vi "Front Panel.vi"() -> ()   [LabVIEW 2020]
uses:
  XControl/Step Control/Step.xctl
  Function/Copy of Function Folder/Function V3.lvlib
panel:
  out "Running?":bool
  in  "Information":string
  in  "File Counter":i32
  in  "Data File Destination":path
  in  "Autorun":bool
  in  "Browser":enum32{"Scan", "Read", "Array"}(tab)
  out "Scan Process Preview":T1(array[cluster]) {"Scan Instrument" items=["Keithley 6430 Scan Voltage", "Dynacool SetField 100Oe", "Dynacool SetPosition", "Dynacool SetTemperature hold", "Dynacool SetTemperature no hold", "Read Time(s)"]}
  out "Read Process Preview":u16[](array[ring]) items=["Keithley 6430 Read Current", "Keithley 6430 Read Voltage", "Dynacool Ch1", "Dynacool Ch2", "Dynacool Ch3", "Dynacool GetField", "Dynacool GetTemperature", "Dynacool GetPosition", "Read Secs"]
  in  "Preview":bool
  in  "Array Preview":string[][](table)
  in  "Step":T2(xcontrol)
  in  "Start":bool
  in  "Load Configuration":bool
  in  "INI File Destination":path
  in  "Read Instrument":i32(listbox)
  in  "Scan Instrument":i32(listbox)
  in  "Initialize":bool
  in  "Quit":bool
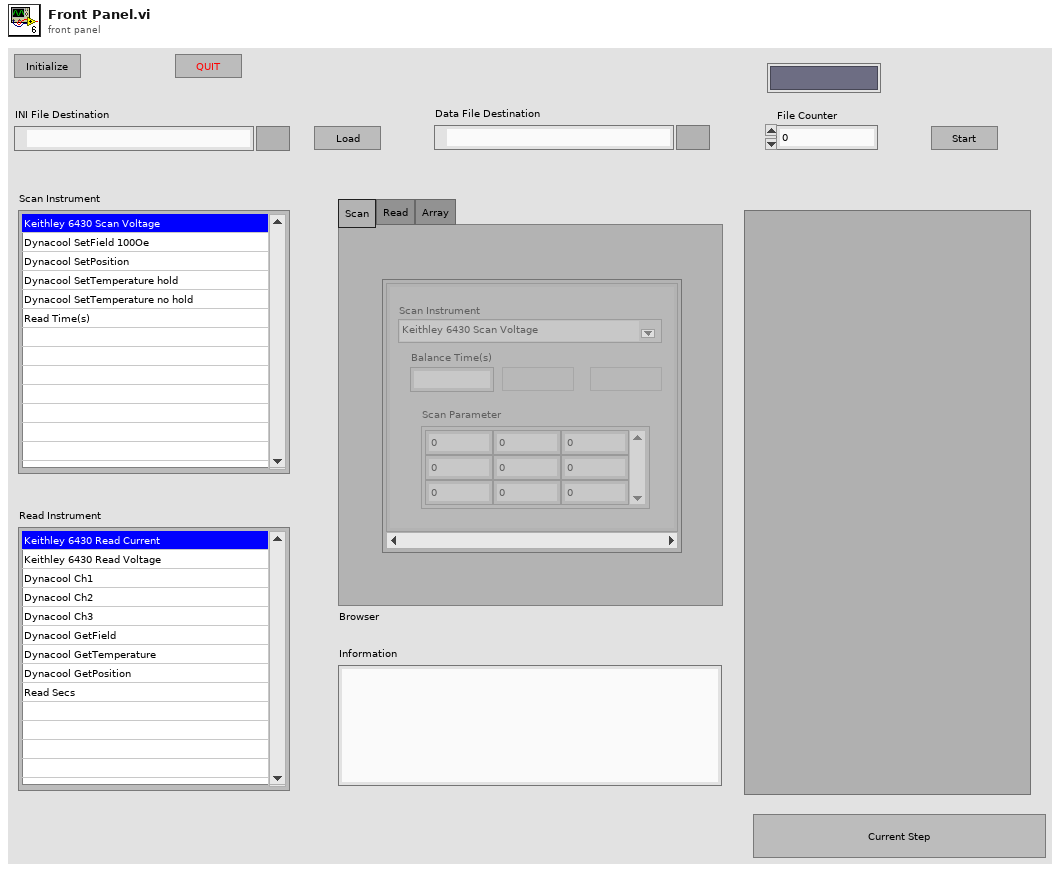
[diagram p1: front panel]
types:
  T1 = cluster{"Scan Instrument":u16, "Linear/Log":bool, "Period/Number":bool, "Balance Time(s)":dbl, "Scan Parameter":dbl[][]}[]
  T2 = cluster{"Wait(s)":dbl, "Interplate Method":u16, "Read Process":u16[], "Scan Process":cluster{"Scan Instrument":u16, "Linear/Log":bool, "Period/Number":bool, "Balance Time(s)":dbl, "Scan Parameter":dbl[][]}[], "Step Information":cluster{"Step Name":string, "Step Description":string}}[]
  T3 = enum16{"Initialize", "Load Configuration", "Preview", "Start", "Shutdown"}
  T4 = cluster{"Wait(s)":dbl, "Interplate Method":u16, "Read Process":u16[], "Scan Process":cluster{"Scan Instrument":u16, "Linear/Log":bool, "Period/Number":bool, "Balance Time(s)":dbl, "Scan Parameter":dbl[][]}[], "Step Information":cluster{"Step Name":string, "Step Description":string}}
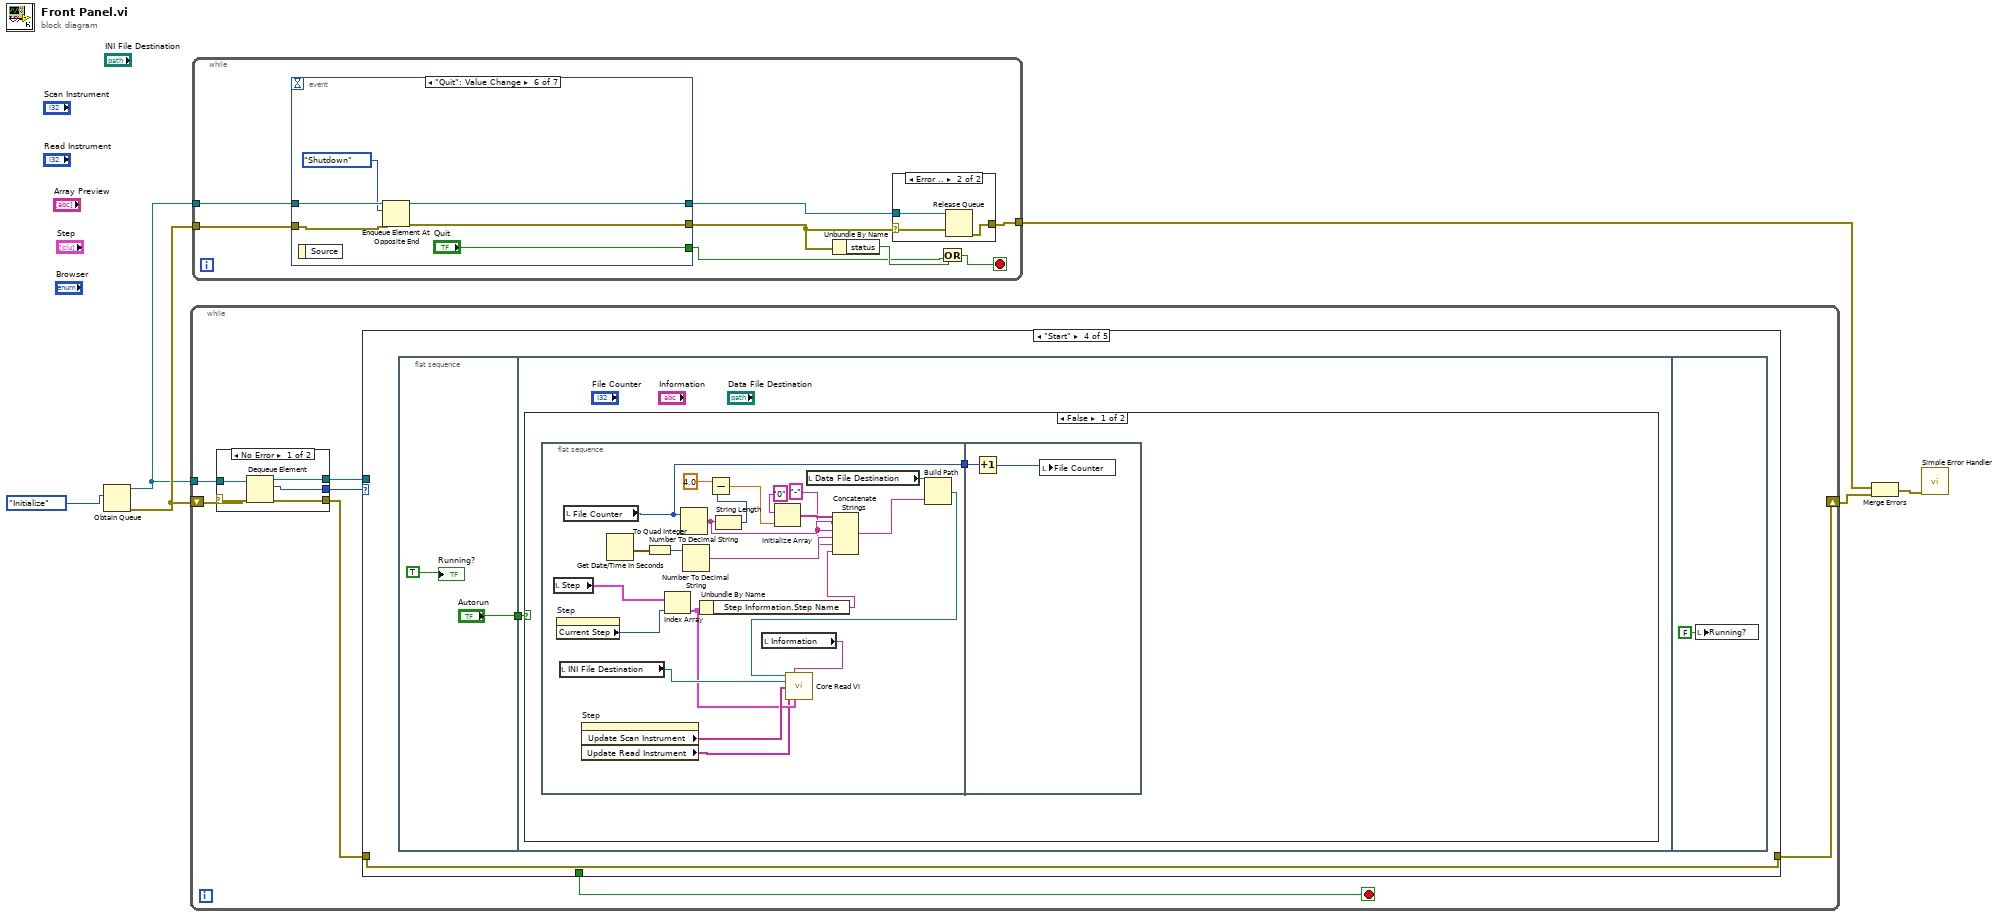
[diagram p0: block diagram]
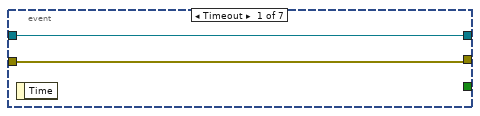
[diagram p3: hidden frame]
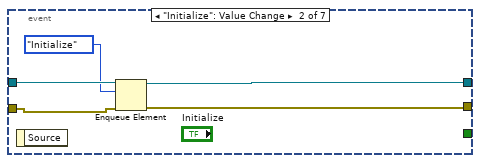
[diagram p4: hidden frame]
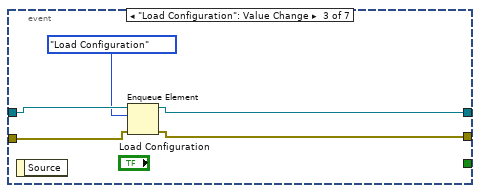
[diagram p5: hidden frame]
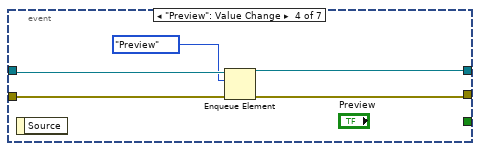
[diagram p6: hidden frame]
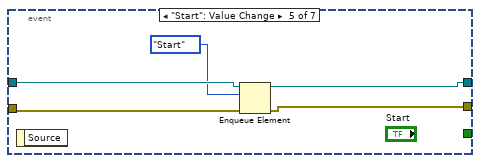
[diagram p7: hidden frame]
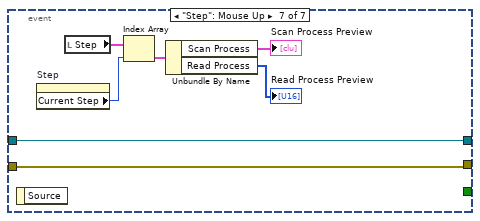
[diagram p8: hidden frame]
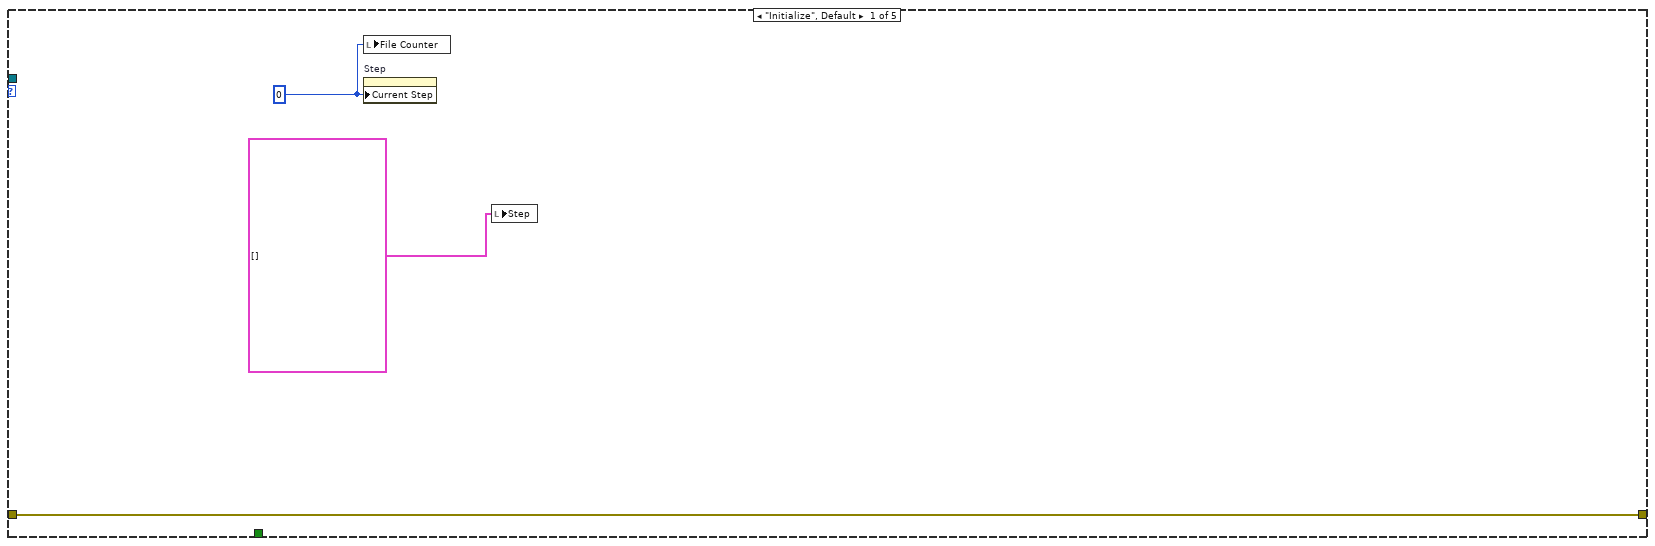
[diagram p9: hidden frame]
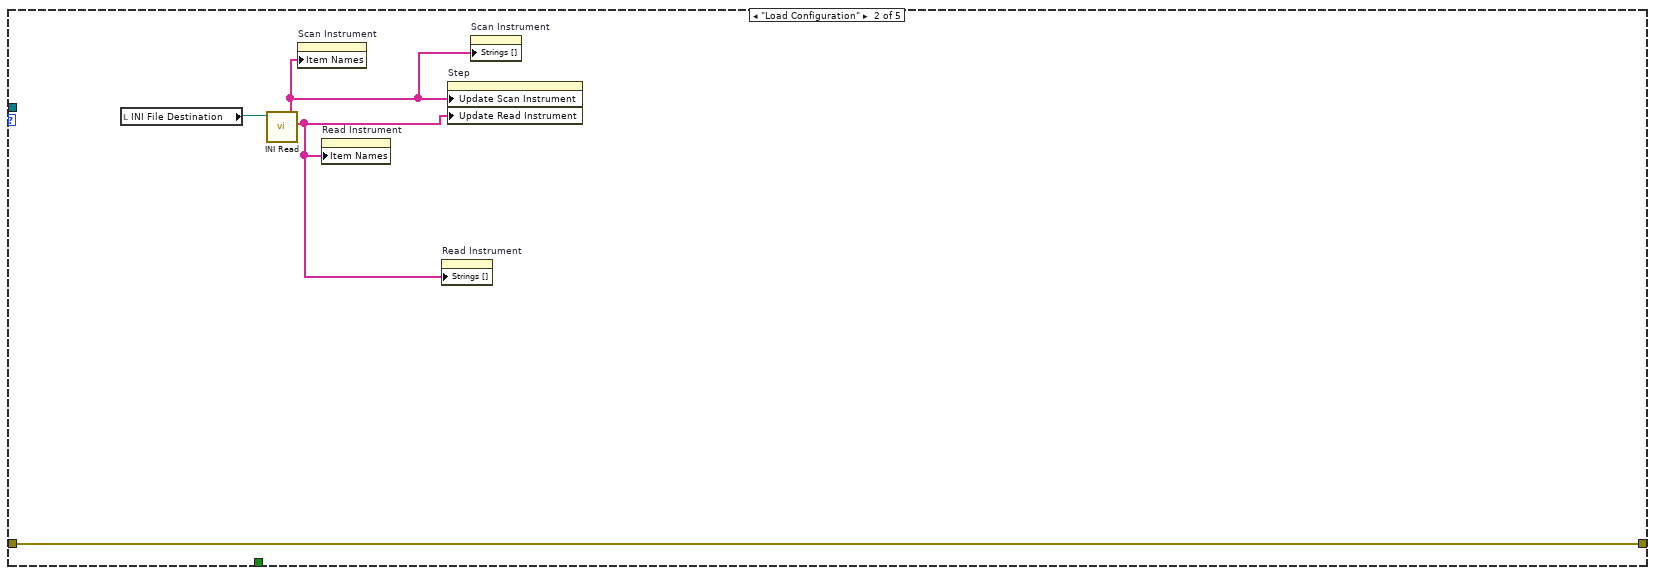
[diagram p10: hidden frame]
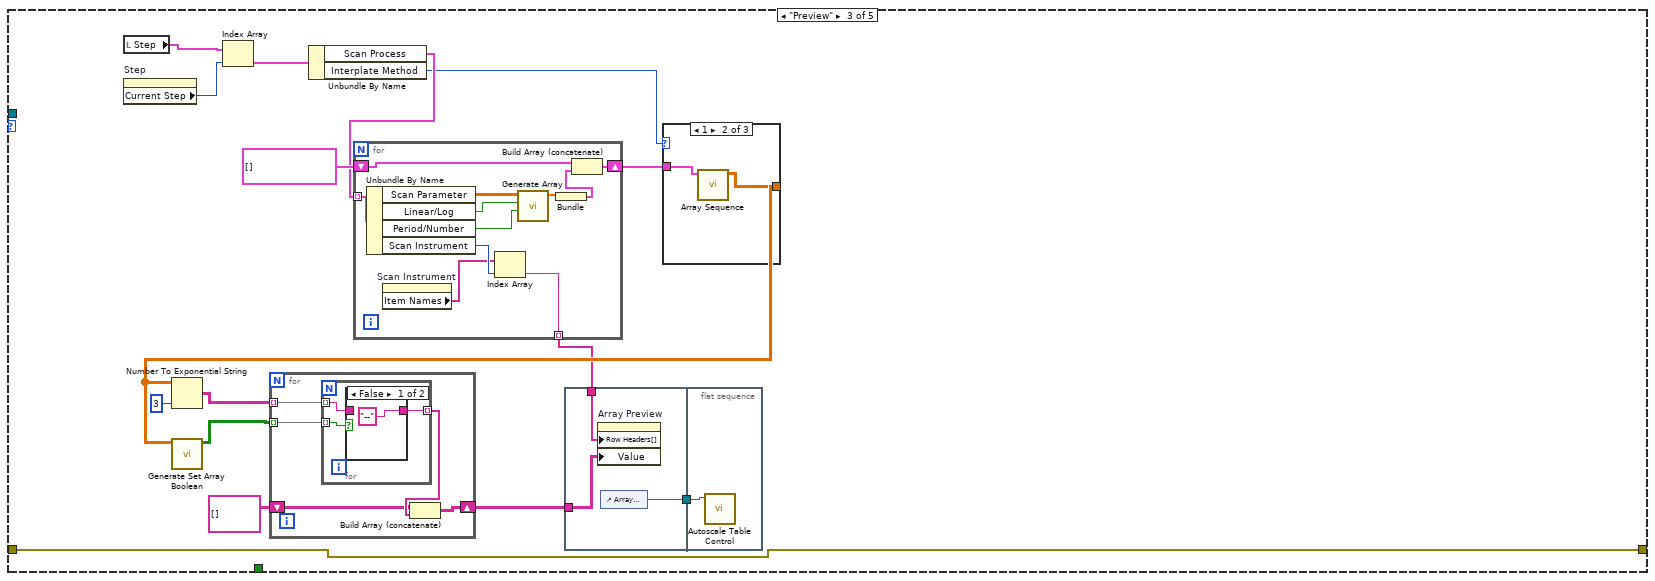
[diagram p11: hidden frame]
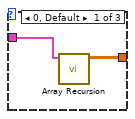
[diagram p13: hidden frame]
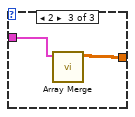
[diagram p14: hidden frame]
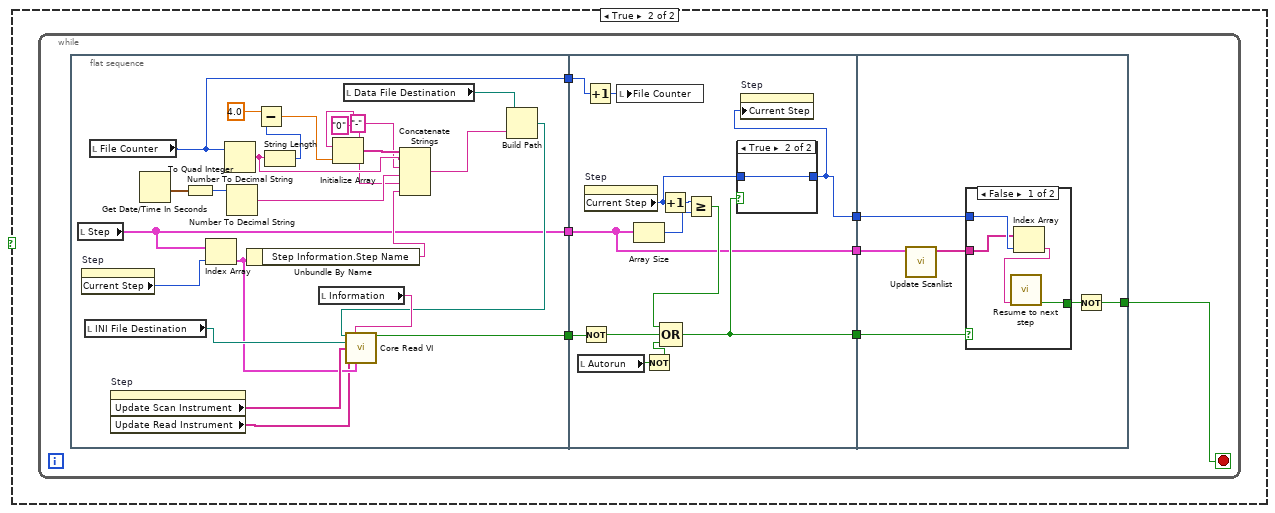
[diagram p15: hidden frame]
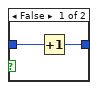
[diagram p16: hidden frame]
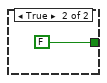
[diagram p17: hidden frame]
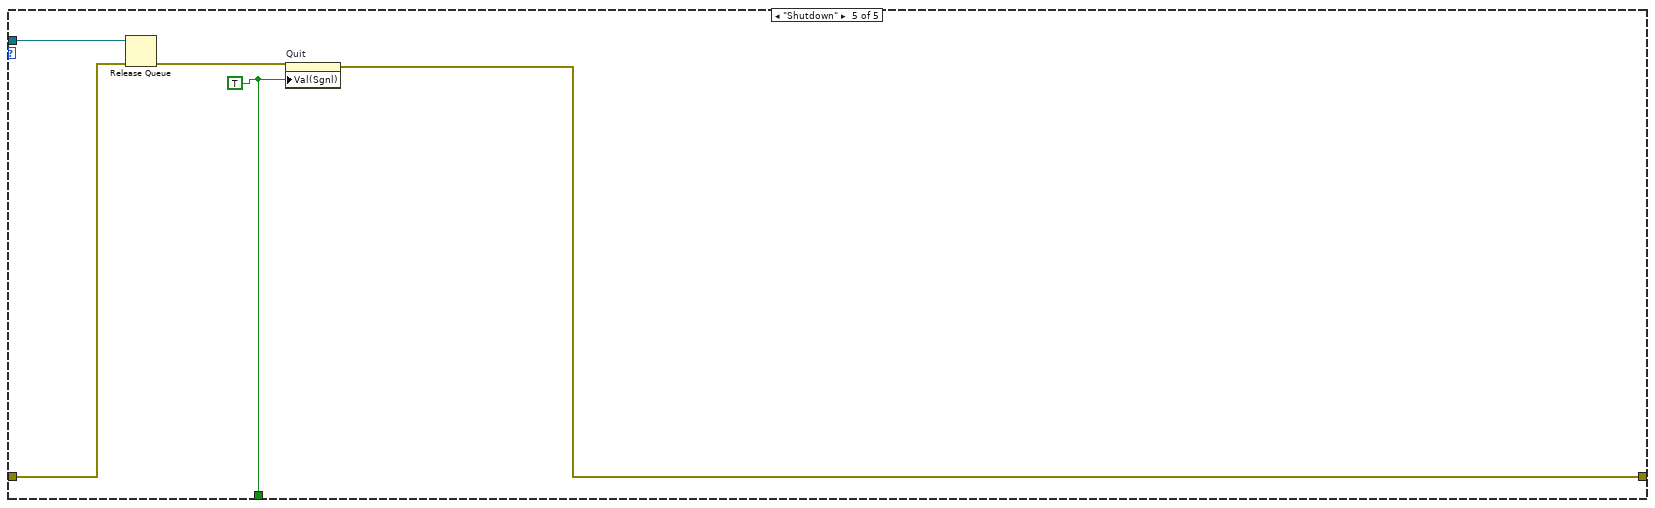
[diagram p18: hidden frame]
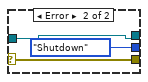
[diagram p19: hidden frame]
diagram:
  n1 = Obtain Queue(element data type=T3."Initialize" ("element")) -> (queue out=w5:refnum<queue>, error out=w6:errorcluster)  [unwired: 4 in, 1 out]
  n2 = while {
    shift-right: [w7] -> w4
    shift-left: w6 -> [w13]
    tunnel: w5 -> [w12]
    stop <- w10 stop-if-true
    n3 = case shown="No Error" w13 {
      selector: w13 -> [w165 w168]
      tunnel: [w164 w168] -> w9
      tunnel: w12 -> [w163 w167]
      tunnel: [w162 w167] -> w11
      tunnel: [w161 T3."Shutdown" ("element")] -> w8
      frame No Error {
        n4 = Dequeue Element(queue=w163, error in (no error)=w165) -> (queue out=w162:refnum<queue>, element=w161:T3, error out=w164:errorcluster)  [unwired: 1 in, 1 out]
      }
      frame Error {
      }
    }
    n5 = case shown="\"Start\"" w8 {
      tunnel: w11 -> [_ _ _ _ w159]
      tunnel: w9 -> [w16 w17 w21 w69 w160]
      tunnel: [w16 w17 w21 w69 w157] -> w7
      tunnel: [_ _ _ _ w156] -> w10
      frame "Initialize", Default {
        w14 = 0 ("Current Step")
        n6 = local write "File Counter"(w14) -> ()
        n7 = property on="Step" class="Step (strict)"("Current Step"=w14) -> ()  [unwired: 2 in, 2 out]
        n8 = local write "Step"(T2 []) -> ()
      }
      frame "Load Configuration" {
        n9 = local read "INI File Destination"() -> (w20:path)
        n10 = call "INI Read.vi"("configuration file path"=w20) -> ("Read Instrument String"=w19:string[], "Scan Instrument String"=w18:string[])  [unwired: 7 in, 2 out]
        n11 = property on="Scan Instrument" class="LstBox (strict)"("Item Names"=w18) -> ()  [unwired: 2 in, 2 out]
        n12 = property on="Read Instrument" class="LstBox (strict)"("Item Names"=w19) -> ()  [unwired: 2 in, 2 out]
        n13 = property on="Read Instrument" class="Ring (strict)"("Strings []"=w19) -> ()  [unwired: 2 in, 2 out]
        n14 = property on="Step" class="Step (strict)"("Update Scan Instrument"=w18, "Update Read Instrument"=w19) -> ()  [unwired: 2 in, 2 out]
        n15 = property on="Scan Instrument" class="Ring (strict)"("Strings []"=w18) -> ()  [unwired: 2 in, 2 out]
      }
      frame "Preview" {
        n16 = local read "Step"() -> (w35:T2)
        n17 = property on="Step" class="Step (strict)"() -> ("Current Step"=w36:i32)  [unwired: 2 in, 2 out]
        n18 = Index Array(array=w35, index=w36) -> (element=w34:T4)
        n19 = Unbundle By Name(w34) -> ("Scan Process"=w32:T1, "Interplate Method"=w31:u16)
        n20 = for {
          tunnel: w32 -> [w67] mode=indexing
          shift-right: [w65] -> w30
          shift-left: cluster{"Output":dbl[]}[] [] -> [w64]
          tunnel: [w62] -> w24 mode=indexing
          n21 = Unbundle By Name(w67) -> ("Scan Parameter"=w60:dbl[][], "Linear/Log"=w59:bool, "Period/Number"=w58:bool, "Scan Instrument"=w63:u16)
          n22 = property on="Scan Instrument" class="LstBox (strict)"() -> ("Item Names"=w57:string[])  [unwired: 2 in, 2 out]
          n23 = Index Array(array=w57, index=w63) -> (element=w62:string)
          n24 = call "Generate Array.vi"("Period/Number"=w58, "Linear/Log"=w59, "Input Array"=w60) -> ("Output"=w61:dbl[])  [unwired: 8 in]
          n25 = Bundle("Output"=w61) -> (w66:cluster{"Output":dbl[]})  [unwired: 1 in]
          n26 = Build Array (concatenate)(w64, w66) -> (w65:cluster{"Output":dbl[]}[])
        }
        n27 = flat-sequence {
          tunnel: w24 -> [w39]
          tunnel: w23 -> [w38]
          tunnel: [w37] -> w22
          tunnel: w22 -> [w40]
          frame #0 {
            n28 = property on="Array Preview" class="Tbl (strict)"("Row Headers[]"=w39, "Value"=w38) -> ()  [unwired: 2 in, 2 out]
            n29 = control-ref of="Array Preview"() -> (w37:refnum<vi>)
          }
          frame #1 {
            n30 = call "Autoscale Table Control.vi"("Input Table Control"=w40) -> ()  [unwired: 10 in, 1 out]
          }
        }
        n31 = case shown="1" w31 {
          tunnel: w30 -> [w52 w54 w56]
          tunnel: [w51 w53 w55] -> w29
          frame 0, Default {
            n32 = call "Array Recursion.vi"("Input Cluster Array"=w52) -> ("Output Array"=w51:dbl[][])  [unwired: 10 in]
          }
          frame 1 {
            n33 = call "Array Sequence.vi"("Input Cluster Array"=w54) -> ("Output Sequence Array"=w53:dbl[][])  [unwired: 10 in]
          }
          frame 2 {
            n34 = call "Array Merge.vi"("Input Cluster Array"=w56) -> ("Output Array"=w55:dbl[][])  [unwired: 10 in]
          }
        }
        n35 = Number To Exponential String(number=w29, precision (6)=i16 3) -> (E-format string=w26:string[][])  [unwired: 2 in]
        n36 = call "Generate Set Array Boolean.vi"("Input Array"=w29) -> ("Output Bool Array"=w25:bool[][])  [unwired: 10 in]
        n37 = for {
          tunnel: w26 -> [w44] mode=indexing
          tunnel: w25 -> [w45] mode=indexing
          shift-right: [w42] -> w23
          shift-left: string[][] [] -> [w41]
          n38 = for {
            tunnel: w45 -> [w48] mode=indexing
            tunnel: w44 -> [w47] mode=indexing
            tunnel: [w46] -> w43 mode=indexing
            n39 = case shown="False" w48 {
              tunnel: w47 -> [_ w50]
              tunnel: ["--" w50] -> w46
              frame False {
              }
              frame True {
              }
            }
          }
          n40 = Build Array (concatenate)(w41, w43) -> (w42:string[][])
        }
      }
      frame "Start" {
        n41 = flat-sequence {
          tunnel: ["Autorun"] -> w68
          tunnel: w68 -> [w72]
          frame #0 {
            "Running?" <- TRUE
          }
          frame #1 {
            n42 = case shown="False" w72 {
              frame False {
                n43 = flat-sequence {
                  tunnel: [w76] -> w73
                  tunnel: w73 -> [w97]
                  frame #0 {
                    w86 = "-"
                    n44 = local read "Step"() -> (w85:T2)
                    n45 = property on="Step" class="Step (strict)"() -> ("Current Step"=w84:i32)  [unwired: 2 in, 2 out]
                    n46 = local read "INI File Destination"() -> (w81:path)
                    n47 = local read "File Counter"() -> (w76:i32)
                    n48 = property on="Step" class="Step (strict)"() -> ("Update Scan Instrument"=w79:string[], "Update Read Instrument"=w77:string[])  [unwired: 2 in, 2 out]
                    n49 = Get Date/Time In Seconds() -> (seconds since 1Jan1904=w89:timestamp)
                    n50 = To Quad Integer(1:w89) -> (0:w88:i64)
                    n51 = Index Array(array=w85, index=w84) -> (element=w78:T4)
                    n52 = Number To Decimal String(number=w76) -> (decimal integer string=w90:string)  [unwired: 1 in]
                    n53 = Number To Decimal String(number=w88) -> (decimal integer string=w87:string)  [unwired: 1 in]
                    n54 = Unbundle By Name(w78) -> ("Step Information.Step Name"=w83:string)
                    n55 = String Length(string=w90) -> (length=w93:i32)
                    n56 = Subtract(x=4.0, y=w93) -> (x-y=w92:dbl)
                    n57 = local read "Information"() -> (w75:string)
                    n58 = Initialize Array("0", w92) -> (w91:string[])
                    n59 = local read "Data File Destination"() -> (w74:path)
                    n60 = Concatenate Strings(w91, w90, w86, w87, w86, w83) -> (w82:string)
                    n61 = Build Path(base path=w74, name or relative path=w82) -> (appended path=w80:path)
                    n62 = call "Core Read VI.vi"("File path"=w80, "Information"=w75, "INI File Destination"=w81, "Update Scan Instrument"=w79, "Update Read Instrument"=w77, "Step Information"=w78) -> ()  [unwired: 9 in, 1 out]
                  }
                  frame #1 {
                    n63 = Increment(x=w97) -> (x+1=w96:i32)
                    n64 = local write "File Counter"(w96) -> ()
                  }
                }
              }
              frame True {
                n65 = while {
                  stop <- w98 stop-if-true
                  n66 = flat-sequence {
                    tunnel: [w107] -> w104
                    tunnel: [w106] -> w103
                    tunnel: [w105] -> w102
                    tunnel: w104 -> [w139]
                    tunnel: w103 -> [w138]
                    tunnel: w102 -> [w131]
                    tunnel: [w133] -> w101
                    tunnel: [w131] -> w100
                    tunnel: [w130] -> w99
                    tunnel: w101 -> [w148]
                    tunnel: w100 -> [w149]
                    tunnel: w99 -> [w146]
                    tunnel: [w144] -> w98
                    frame #0 {
                      w111 = "-"
                      n67 = local read "Step"() -> (w105:T2)
                      n68 = property on="Step" class="Step (strict)"() -> ("Current Step"=w120:i32)  [unwired: 2 in, 2 out]
                      n69 = local read "INI File Destination"() -> (w117:path)
                      n70 = local read "File Counter"() -> (w107:i32)
                      n71 = property on="Step" class="Step (strict)"() -> ("Update Scan Instrument"=w116:string[], "Update Read Instrument"=w114:string[])  [unwired: 2 in, 2 out]
                      n72 = Get Date/Time In Seconds() -> (seconds since 1Jan1904=w123:timestamp)
                      n73 = To Quad Integer(1:w123) -> (0:w122:i64)
                      n74 = Index Array(array=w105, index=w120) -> (element=w115:T4)
                      n75 = Number To Decimal String(number=w107) -> (decimal integer string=w124:string)  [unwired: 1 in]
                      n76 = Number To Decimal String(number=w122) -> (decimal integer string=w121:string)  [unwired: 1 in]
                      n77 = Unbundle By Name(w115) -> ("Step Information.Step Name"=w119:string)
                      n78 = String Length(string=w124) -> (length=w127:i32)
                      n79 = Subtract(x=4.0, y=w127) -> (x-y=w126:dbl)
                      n80 = local read "Information"() -> (w113:string)
                      n81 = Initialize Array("0", w126) -> (w125:string[])
                      n82 = local read "Data File Destination"() -> (w112:path)
                      n83 = Concatenate Strings(w125, w124, w111, w121, w111, w119) -> (w118:string)
                      n84 = Build Path(base path=w112, name or relative path=w118) -> (appended path=w108:path)
                      n85 = call "Core Read VI.vi"("File path"=w108, "Information"=w113, "INI File Destination"=w117, "Update Scan Instrument"=w116, "Update Read Instrument"=w114, "Step Information"=w115) -> ("Continue?"=w106:bool)  [unwired: 9 in]
                    }
                    frame #1 {
                      n86 = local read "Autorun"() -> (w129:bool)
                      n87 = Not(x=w138) -> (.not. x?=w137:bool)
                      n88 = Increment(x=w139) -> (x+1=w140:i32)
                      n89 = property on="Step" class="Step (strict)"() -> ("Current Step"=w132:i32)  [unwired: 2 in, 2 out]
                      n90 = local write "File Counter"(w140) -> ()
                      n91 = Array Size(array=w131) -> (size(s)=w135:i32)
                      n92 = Not(x=w129) -> (.not. x?=w128:bool)
                      n93 = Increment(x=w132) -> (x+1=w136:i32)
                      n94 = Greater Or Equal?(x=w136, y=w135) -> (x >= y?=w134:bool)
                      n95 = Compound Arithmetic op=OR(w134, w137, w128) -> (w133:bool)
                      n96 = case shown="True" w133 {
                        tunnel: w132 -> [w142 w143]
                        tunnel: [w141 w143] -> w130
                        frame False {
                          n97 = Increment(x=w142) -> (x+1=w141:i32)
                        }
                        frame True {
                        }
                      }
                      n98 = property on="Step" class="Step (strict)"("Current Step"=w130) -> ()  [unwired: 2 in, 2 out]
                    }
                    frame #2 {
                      n99 = call "Update Scanlist.vi"("Step"=w149) -> ("Scan List"=w147:string[])  [unwired: 10 in]
                      n100 = case shown="False" w148 {
                        tunnel: [w150 FALSE] -> w145
                        tunnel: w147 -> [w152 _]
                        tunnel: w146 -> [w153 _]
                        frame False {
                          n101 = Index Array(array=w152, index=w153) -> (element=w151:string)
                          n102 = call "Resume to next step.vi"("Next Step Name"=w151) -> ("Continue?"=w150:bool)  [unwired: 10 in]
                        }
                        frame True {
                        }
                      }
                      n103 = Not(x=w145) -> (.not. x?=w144:bool)
                    }
                  }
                }
              }
            }
          }
          frame #2 {
            n104 = local write "Running?"(FALSE) -> ()
          }
        }
      }
      frame "Shutdown" {
        w156 = TRUE
        n105 = Release Queue(queue=w159, error in (no error)=w160) -> (error out=w158:errorcluster)  [unwired: 1 in, 2 out]
        n106 = property on="Quit" class="Bool (strict)"(error in=w158, "Val(Sgnl)"=w156) -> (error out=w157:errorcluster)  [unwired: 1 in, 1 out]
      }
    }
  }
  n107 = while {
    tunnel: w6 -> [w176]
    tunnel: w5 -> [w175]
    tunnel: [w169] -> w3
    stop <- w173 stop-if-true
    n108 = event shown="[5] \"Quit\": Value Change" {
      selector: _ -> [_ _ _ _ _ _ _]
      dyn-events: _ -> [_ _ _ _ _ _ _]
      timeout: _ -> [_ _ _ _ _ _ _]
      tunnel: [_ _ _ _ _ "Quit" _] -> w171
      tunnel: w176 -> [w181 w187 w192 w197 w202 w207 w209]
      tunnel: [w181 w186 w191 w196 w201 w206 w209] -> w174
      tunnel: w175 -> [w182 w185 w190 w194 w200 w205 w210]
      tunnel: [w182 w184 w189 w195 w199 w204 w210] -> w170
      event Timeout {
        n109 = event-data() -> ()  [unwired: 1 in, 1 out]
      }
      event "Initialize": Value Change {
        n110 = event-data() -> ()  [unwired: 1 in, 1 out]
        n111 = Enqueue Element(queue=w185, element=T3."Initialize", error in (no error)=w187) -> (queue out=w184:refnum<queue>, error out=w186:errorcluster)  [unwired: 1 in, 1 out]
      }
      event "Load Configuration": Value Change {
        n112 = event-data() -> ()  [unwired: 1 in, 1 out]
        n113 = Enqueue Element(queue=w190, element=T3."Load Configuration", error in (no error)=w192) -> (queue out=w189:refnum<queue>, error out=w191:errorcluster)  [unwired: 1 in, 1 out]
      }
      event "Preview": Value Change {
        n114 = event-data() -> ()  [unwired: 1 in, 1 out]
        n115 = Enqueue Element(queue=w194, element=T3."Preview", error in (no error)=w197) -> (queue out=w195:refnum<queue>, error out=w196:errorcluster)  [unwired: 1 in, 1 out]
      }
      event "Start": Value Change {
        n116 = event-data() -> ()  [unwired: 1 in, 1 out]
        n117 = Enqueue Element(queue=w200, element=T3."Start", error in (no error)=w202) -> (queue out=w199:refnum<queue>, error out=w201:errorcluster)  [unwired: 1 in, 1 out]
      }
      event "Quit": Value Change {
        n118 = event-data() -> ()  [unwired: 1 in, 1 out]
        n119 = Enqueue Element At Opposite End(queue=w205, element=T3."Shutdown", error in (no error)=w207) -> (queue out=w204:refnum<queue>, error out=w206:errorcluster)  [unwired: 1 in, 1 out]
      }
      event "Step": Mouse Up {
        n120 = event-data() -> ()  [unwired: 1 in, 1 out]
        n121 = property on="Step" class="Step (strict)"() -> ("Current Step"=w214:i32)  [unwired: 2 in, 2 out]
        n122 = local read "Step"() -> (w215:T2)
        n123 = Index Array(array=w215, index=w214) -> (element=w213:T4)
        n124 = Unbundle By Name(w213) -> ("Scan Process"=→"Scan Process Preview":T1, "Read Process"=→"Read Process Preview":u16[])
      }
    }
    n125 = Unbundle By Name(w174) -> ("status"=w172:bool)
    n126 = case shown="Error .." w174 {
      selector: w174 -> [w177 w178]
      tunnel: w170 -> [_ w180]
      tunnel: [w177 w179] -> w169
      frame No Error {
      }
      frame Error {
        n127 = Release Queue(queue=w180, error in (no error)=w178) -> (error out=w179:errorcluster)  [unwired: 1 in, 2 out]
      }
    }
    n128 = Or(x=w172, y=w171) -> (x .or. y?=w173:bool)
  }
  n129 = Merge Errors(w3, w4) -> (w2:errorcluster)
  n130 = call <vilib>:"Simple Error Handler.vi"("error in (no error)"=w2) -> ()  [unwired: 4 in, 5 out]
